vi "Test MCP4725 2.vi"() -> ()   [LabVIEW 2014]
uses:
  <vilib>/LabVIEW Universal Transcriptor/MCP4725/MCP4725.lvclass
  <vilib>/LabVIEW Universal Transcriptor/LabVIEW for Arduino Math Library/Arduino Math.lvlib
panel:
  in  "signal type":T1(ring)=enum."user defined 2"
  out "MCP4725 out":refnum<class "MCP4725.lvclass">
  out "error out":errorcluster
  in  "Error In":errorcluster
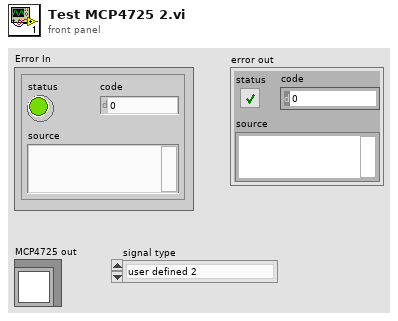
[diagram p1: front panel]
types:
  T1 = enum16{"triangle", "square", "user defined", "feedback gen.", "user defined 2"}
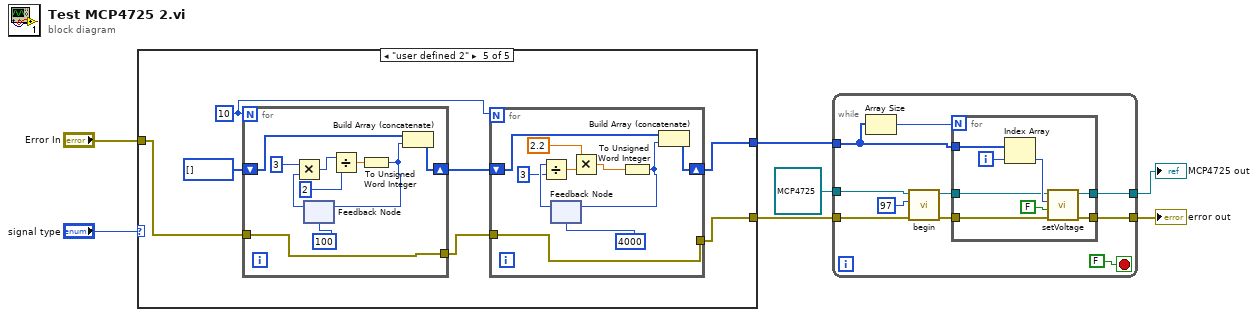
[diagram p0: block diagram]
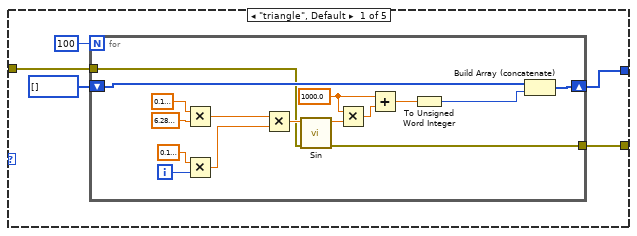
[diagram p2: hidden frame]
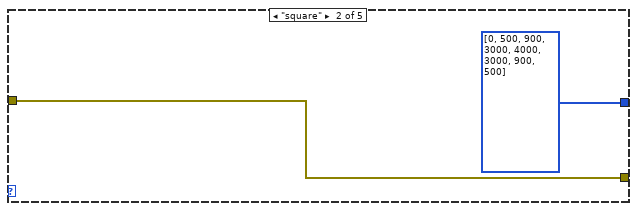
[diagram p3: hidden frame]
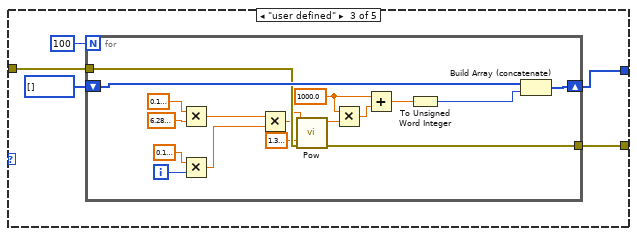
[diagram p4: hidden frame]
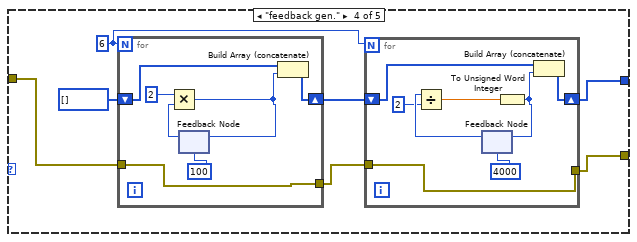
[diagram p5: hidden frame]
diagram:
  n1 = case shown="\"user defined 2\"" "signal type" {
    tunnel: [w8 u16[] [0, 500, 900, 3000, 4000, 3000, 900, 500] w31 w56 w75] -> w4
    tunnel: "Error In" -> [w10 w29 w33 w55 w77]
    tunnel: [w9 w29 w32 w53 w76] -> w2
    frame "triangle", Default {
      n2 = for {
        N: 100 -> [_]
        tunnel: [w16] -> w9
        shift-right: [w17] -> w8
        shift-left: u16[] [] -> [w18]
        tunnel: w10 -> [w13]
        i -> [w25]
        w19 = sgl 1000.0 ("x")
        n3 = Multiply(x=sgl 0.1, y=sgl 6.28 ("x")) -> (x*y=w26:sgl)
        n4 = Multiply(x=sgl 0.1, y=w25) -> (x*y=w23:sgl)
        n5 = Multiply(x=w26, y=w23) -> (x*y=w22:sgl)
        n6 = call <vilib>:"Sin.vi"("Error In"=w13, "x"=w22) -> ("Error Out"=w16:errorcluster, "sin(x)"=w21:sgl)  [unwired: 8 in]
        n7 = Multiply(x=w19, y=w21) -> (x*y=w20:sgl)
        n8 = Add(x=w19, y=w20) -> (x+y=w15:sgl)
        n9 = To Unsigned Word Integer(number=w15) -> (unsigned 16bit integer=w14:u16)
        n10 = Build Array (concatenate)(w18, w14) -> (w17:u16[])
      }
    }
    frame "square" {
    }
    frame "user defined" {
      n11 = for {
        N: 100 -> [_]
        tunnel: [w41] -> w32
        shift-right: [w42] -> w31
        shift-left: u16[] [] -> [w43]
        tunnel: w33 -> [w38]
        i -> [w49]
        w44 = sgl 1000.0 ("x")
        n12 = Multiply(x=sgl 0.1, y=sgl 6.28 ("x")) -> (x*y=w50:sgl)
        n13 = Multiply(x=sgl 0.1, y=w49) -> (x*y=w47:sgl)
        n14 = Multiply(x=w50, y=w47) -> (x*y=w37:sgl)
        n15 = call <vilib>:"Pow.vi"("Error In"=w38, "y"=sgl 1.4, "x"=w37) -> ("Error Out"=w41:errorcluster, "pow(x,y)"=w46:sgl)  [unwired: 7 in]
        n16 = Multiply(x=w44, y=w46) -> (x*y=w45:sgl)
        n17 = Add(x=w44, y=w45) -> (x+y=w40:sgl)
        n18 = To Unsigned Word Integer(number=w40) -> (unsigned 16bit integer=w39:u16)
        n19 = Build Array (concatenate)(w43, w39) -> (w42:u16[])
      }
    }
    frame "feedback gen." {
      w58 = 6
      n20 = for {
        N: w58 -> [_]
        shift-right: [w69] -> w57
        shift-left: u16[] [] -> [w70]
        tunnel: w55 -> [w68]
        tunnel: [w68] -> w54
        n21 = feedback #1(u16 100) -> (w73:u16)
        n22 = Multiply(x=u16 2, y=w73) -> (x*y=w71:u16)
        n23 = feedback-in #1(w71) -> ()
        n24 = Build Array (concatenate)(w70, w71) -> (w69:u16[])
      }
      n25 = for {
        N: w58 -> [_]
        shift-right: [w64] -> w56
        shift-left: w57 -> [w65]
        tunnel: w54 -> [w60]
        tunnel: [w60] -> w53
        n26 = feedback #2(u16 4000) -> (w62:u16)
        n27 = Divide(x=w62, y=u16 2) -> (x/y=w66:dbl)
        n28 = To Unsigned Word Integer(number=w66) -> (unsigned 16bit integer=w63:u16)
        n29 = feedback-in #2(w63) -> ()
        n30 = Build Array (concatenate)(w65, w63) -> (w64:u16[])
      }
    }
    frame "user defined 2" {
      w80 = 10
      n31 = for {
        N: w80 -> [_]
        shift-right: [w97] -> w79
        shift-left: u16[] [] -> [w98]
        tunnel: w77 -> [w96]
        tunnel: [w96] -> w78
        n32 = feedback #3(u16 100) -> (w100:u16)
        n33 = Multiply(x=u16 3, y=w100) -> (x*y=w95:u16)
        n34 = Divide(x=w95, y=u16 2) -> (x/y=w93:dbl)
        n35 = To Unsigned Word Integer(number=w93) -> (unsigned 16bit integer=w92:u16)
        n36 = feedback-in #3(w92) -> ()
        n37 = Build Array (concatenate)(w98, w92) -> (w97:u16[])
      }
      n38 = for {
        N: w80 -> [_]
        shift-right: [w89] -> w75
        shift-left: w79 -> [w90]
        tunnel: w78 -> [w85]
        tunnel: [w85] -> w76
        n39 = feedback #4(u16 4000) -> (w87:u16)
        n40 = Divide(x=w87, y=u16 3) -> (x/y=w84:dbl)
        n41 = Multiply(x=2.2, y=w84) -> (x*y=w82:dbl)
        n42 = To Unsigned Word Integer(number=w82) -> (unsigned 16bit integer=w88:u16)
        n43 = feedback-in #4(w88) -> ()
        n44 = Build Array (concatenate)(w90, w88) -> (w89:u16[])
      }
    }
  }
  n45 = while {
    tunnel: w2 -> [w111]
    tunnel: refnum<class "MCP4725.lvclass"> refnum ("MCP4725 in") -> [w109]
    tunnel: w4 -> [w107]
    tunnel: [w104] -> w5
    tunnel: [w103] -> w6
    stop <- FALSE stop-if-true
    n46 = Array Size(array=w107) -> (size(s)=w108:i32)
    n47 = call <vilib>:"begin.vi"("error in (no error)"=w111, "I2C addr"=u8 97, "MCP4725 in"=w109) -> ("error out"=w106:errorcluster, "MCP4725 out"=w105:refnum<class "MCP4725.lvclass">)  [unwired: 7 in]
    n48 = for {
      N: w108 -> [_]
      tunnel: w107 -> [w118]
      tunnel: w106 -> [w115]
      tunnel: [w114] -> w103
      tunnel: w105 -> [w113]
      tunnel: [w112] -> w104
      i -> [w119]
      n49 = Index Array(array=w118, index=w119) -> (element=w117:u16)
      n50 = call <vilib>:"setVoltage.vi"("error in (no error)"=w115, "writeEEPROM?"=FALSE, "voltage"=w117, "MCP4725 in"=w113) -> ("error out"=w114:errorcluster, "MCP4725 out"=w112:refnum<class "MCP4725.lvclass">)  [unwired: 6 in]
    }
  }
  "error out" <- w6
  "MCP4725 out" <- w5
